vi "Read Spectrum Continuously.vi"() -> ()   [LabVIEW 2021]
uses:
  <vilib>/Utility/error.llb/DialogType.ctl
panel:
  out "Spectrum number":i32
  out "Read time (ms)":u32
  in  "Ref Level Auto":bool
  out "Min":dbl
  out "Sec":dbl
  out "H":dbl
  in  "Stop Button":bool
  out "P x Lambda Graph":cluster{dbl[], dbl[]}(graph)
  out "Corrente Atual (mA)":dbl
  out "P x I Graph":cluster{dbl[], dbl[]}(graph)
  in  "Start Button":bool
  in  "Cluster de Dados de Entrada":T1={"Corrente Inicial (mA)"=150.0, "Limite de Temperatura"=27.0, "Temperatura"=25.0, "Corrente Limite (mA)"=300, "Centralizar pico (nm)"=1550.0, "Valor de Span (nm)"=200.0, "Passo (mA)"=0.0, "Corrente Final (mA)"=150.0, "Resolucao"=enum."High", "Modo"=enum."Laser"} {"Corrente Final (mA)" min=0.0 step=1.0; "Passo (mA)" min=1.0 step=1.0; "Valor de Span (nm)" min=0.1 max=1400.0 format="%.2f"; "Centralizar pico (nm)" format="%.2f"; "Temperatura" min=-100.0 max=199.9 step=0.1; "Limite de Temperatura" min=-100.0 max=199.9 step=0.1; "Corrente Inicial (mA)" min=0.0 step=1.0}
  out "XY Graph":T2(graph)
  in  "Pasta Destino":path=path "d:/Users/acquisition"
  in  "GPIB Analisador de Espectros":refnum<visa-resource-name>="GPIB0::8::INSTR"
  in  "error in (no error)":errorcluster
  out "error out":errorcluster
  # "Tempo Gasto"
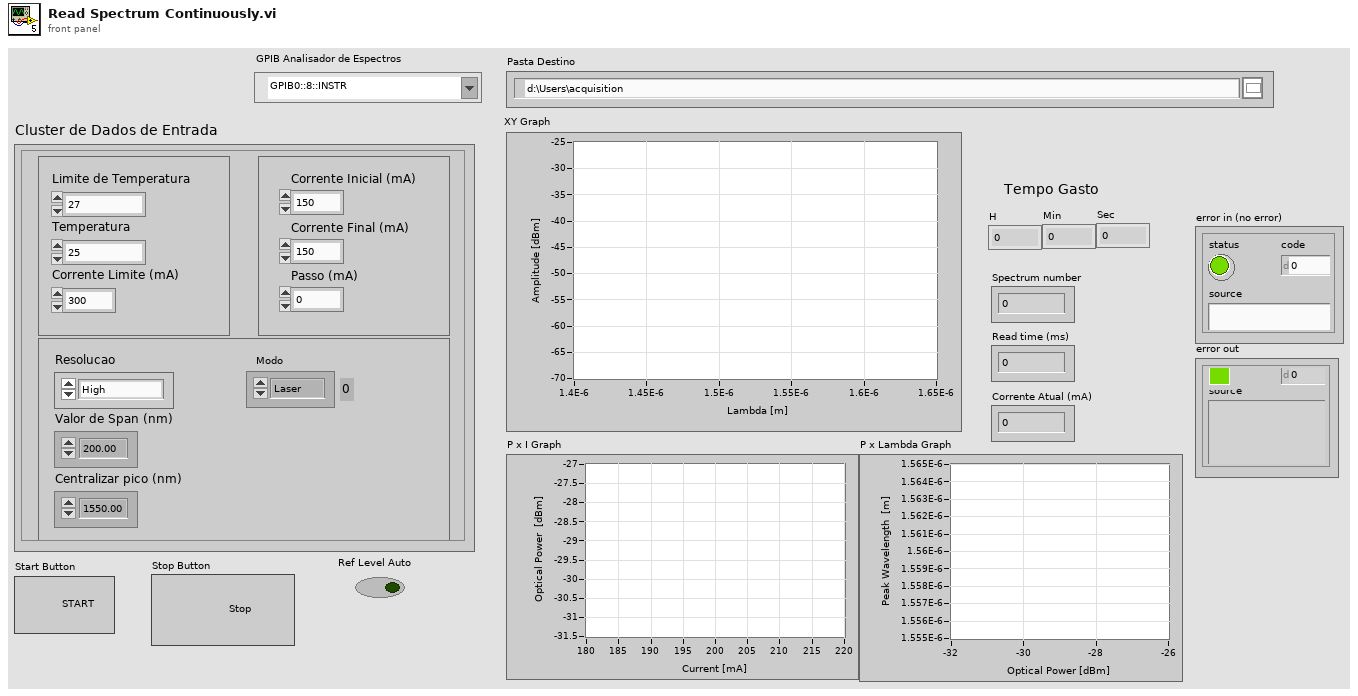
[diagram p1: front panel]
types:
  T1 = cluster{"Corrente Inicial (mA)":dbl, "Limite de Temperatura":dbl, "Temperatura":dbl, "Corrente Limite (mA)":i32, "Centralizar pico (nm)":dbl, "Valor de Span (nm)":dbl, "Passo (mA)":dbl, "Corrente Final (mA)":dbl, "Resolucao":enum16{"Normal", "High"}, "Modo":enum16{"Laser", "Led"}}
  T2 = cluster{"Wavelike Data":dbl[], "Wavelike Data":dbl[]}
  T3 = typedef "DialogType.ctl" = u16
  T4 = cluster{"Limite de Temperatura":dbl, "Temperatura":dbl, "Corrente Inicial (mA)":dbl, "Corrente Limite (mA)":i32, "Resolucao":enum16{"Normal", "High"}, "Centralizar pico (nm)":dbl, "Valor de Span (nm)":dbl, "Modo":enum16{"Laser", "Led"}}
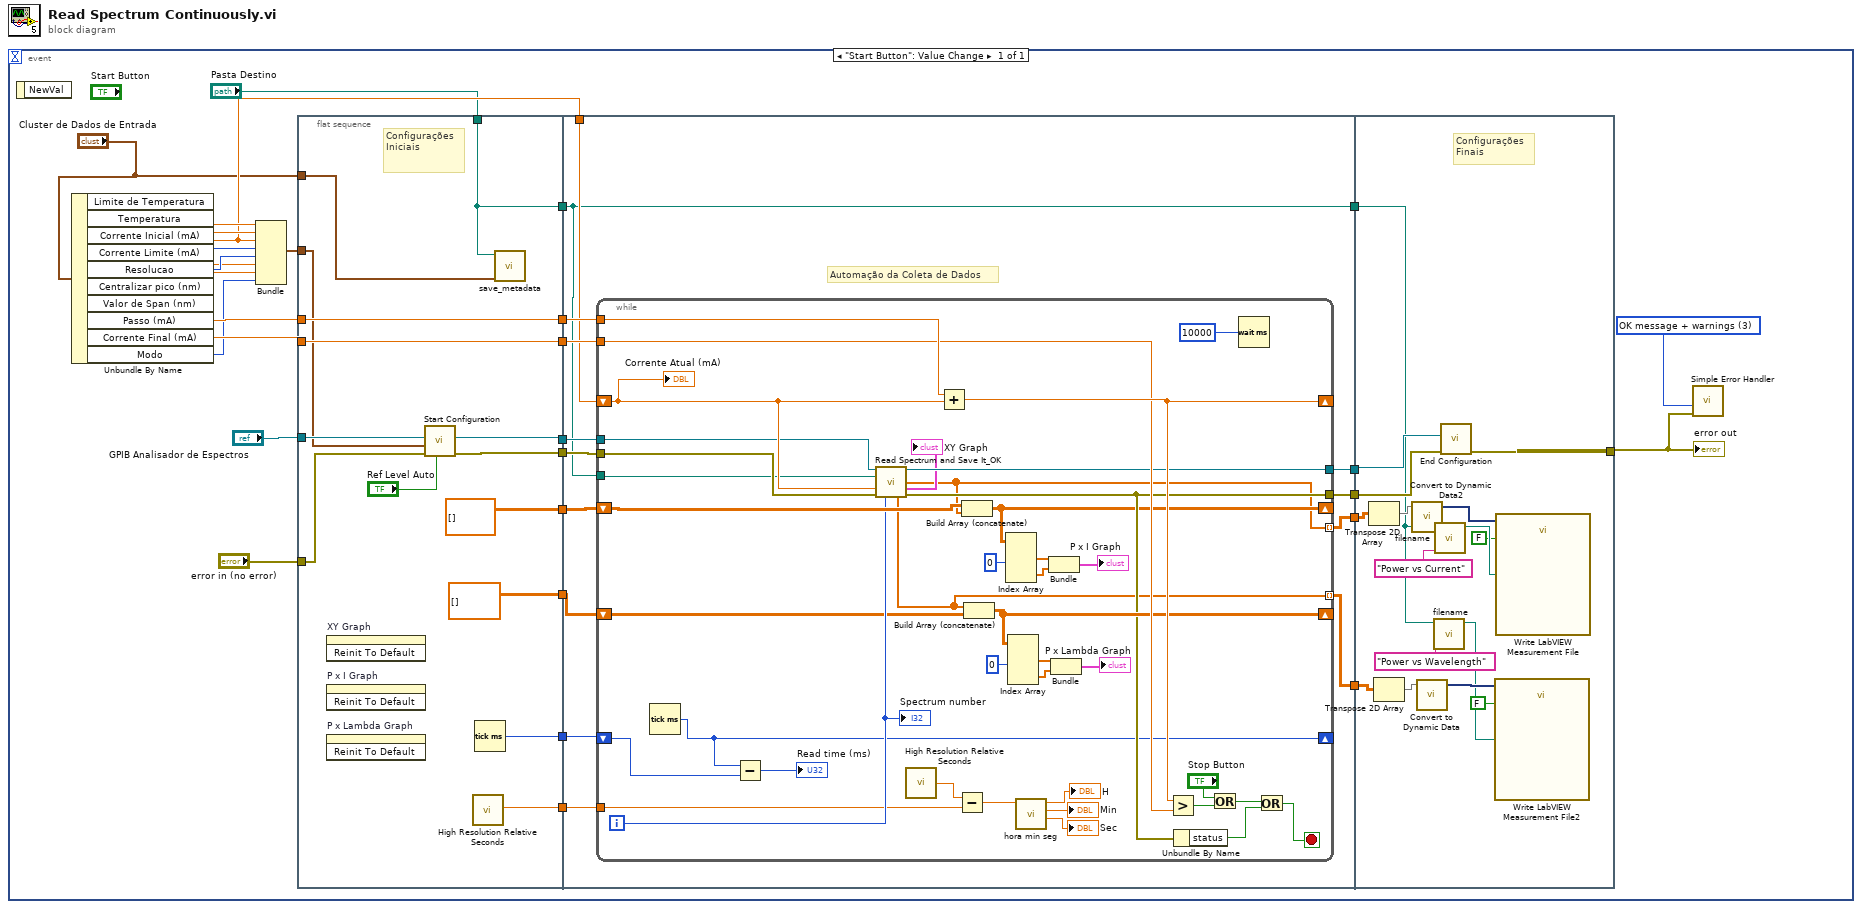
[diagram p0: block diagram]
diagram:
  n1 = event shown="[0] \"Start Button\": Value Change" {
    selector: _ -> [_]
    dyn-events: _ -> [_]
    timeout: _ -> [_]
    event "Start Button": Value Change {
      w11 = T3 3 items=["no dialog", "OK message", "continue or stop message", "OK message + warnings", "continue/stop + warnings"] ("type of dialog (OK msg:1)")
      n2 = event-data() -> ()  [unwired: 1 in, 1 out]
      n3 = Unbundle By Name("Cluster de Dados de Entrada") -> ("Limite de Temperatura"=w25:dbl, "Temperatura"=w24:dbl, "Corrente Inicial (mA)"=w16:dbl, "Corrente Limite (mA)"=w23:i32, "Resolucao"=w22:enum16{"Normal", "High"}, "Centralizar pico (nm)"=w21:dbl, "Valor de Span (nm)"=w19:dbl, "Passo (mA)"=w18:dbl, "Corrente Final (mA)"=w17:dbl, "Modo"=w5:enum16{"Laser", "Led"})
      n4 = Bundle("Limite de Temperatura"=w25, "Temperatura"=w24, "Corrente Inicial (mA)"=w16, "Corrente Limite (mA)"=w23, "Resolucao"=w22, "Centralizar pico (nm)"=w21, "Valor de Span (nm)"=w19, "Modo"=w5) -> (w20:T4)  [unwired: 1 in]
      n5 = flat-sequence {
        tunnel: "error in (no error)" -> [w39]
        tunnel: [w45] -> w31
        tunnel: "GPIB Analisador de Espectros" -> [w44]
        tunnel: [w43] -> w30
        tunnel: [w42] -> w29
        tunnel: w18 -> [w42]
        tunnel: w17 -> [w41]
        tunnel: [w41] -> w28
        tunnel: w20 -> [w36]
        tunnel: [dbl[][] []] -> w15
        tunnel: [dbl[][] []] -> w10
        tunnel: "Cluster de Dados de Entrada" -> [w33]
        tunnel: [w35] -> w4
        tunnel: [w34] -> w3
        tunnel: [w32] -> w2
        tunnel: "Pasta Destino" -> [w32]
        tunnel: w31 -> [w59]
        tunnel: w30 -> [w58]
        tunnel: w29 -> [w57]
        tunnel: w28 -> [w56]
        tunnel: w16 -> [w55]
        tunnel: w15 -> [w54]
        tunnel: [w53] -> w14
        tunnel: [w52] -> w13
        tunnel: w10 -> [w51]
        tunnel: [w46] -> w9
        tunnel: [w50] -> w8
        tunnel: [w49] -> w7
        tunnel: w4 -> [w48]
        tunnel: w3 -> [w47]
        tunnel: w2 -> [w46]
        tunnel: [w115] -> w12
        tunnel: w14 -> [w114]
        tunnel: w13 -> [w113]
        tunnel: w9 -> [w102]
        tunnel: w8 -> [w104]
        tunnel: w7 -> [w106]
        frame #0 {
          # "Configurações\nIniciais"
          n6 = invoke on="XY Graph" class="XYGraph (strict)" method="Reinit To Default"() -> ()  [unwired: 3 in, 3 out]
          n7 = invoke on="P x I Graph" class="XYGraph (strict)" method="Reinit To Default"() -> ()  [unwired: 3 in, 3 out]
          n8 = invoke on="P x Lambda Graph" class="XYGraph (strict)" method="Reinit To Default"() -> ()  [unwired: 3 in, 3 out]
          n9 = call "Start Configuration.vi"("Ref Lvl Auto"="Ref Level Auto", "error in (no error)"=w39, "Cluster de Dados"=w36, "GPIB Espectrometro"=w44) -> ("error out"=w45:errorcluster, "Spectrometer out"=w43:refnum<visa-resource-name>)  [unwired: 6 in]
          n10 = call <vilib>:"High Resolution Relative Seconds.vi"() -> ("relative seconds"=w34:dbl)
          n11 = Tick Count (ms)() -> (millisecond timer value=w35:u32)
          n12 = call "save_metadata.vi"("Cluster de Dados de Entrada"=w33, "Pasta Destino"=w32) -> ()  [unwired: 10 in]
        }
        frame #1 {
          # "Automação da Coleta de Dados"
          n13 = while {
            shift-right: [w97] -> _
            shift-left: w55 -> [w98]
            tunnel: w59 -> [w91]
            tunnel: w58 -> [w96]
            tunnel: w57 -> [w95]
            tunnel: w56 -> [w94]
            shift-right: [w69] -> _
            shift-left: w54 -> [w90]
            tunnel: [w79] -> w53
            tunnel: [w85] -> w52
            shift-right: [w80] -> _
            shift-left: w51 -> [w81]
            tunnel: w46 -> [w70]
            tunnel: [w68] -> w50 mode=indexing
            tunnel: [w67] -> w49 mode=indexing
            shift-right: [w64] -> _
            shift-left: w48 -> [w66]
            tunnel: w47 -> [w62]
            i -> [w86]
            stop <- w77 stop-if-true
            n14 = Tick Count (ms)() -> (millisecond timer value=w64:u32)
            n15 = Subtract(x=w64, y=w66) -> (x-y=→"Read time (ms)":u32)
            n16 = call "Read Spectrum and Save It_OK.vi"("VISA Session"=w96, "Pasta Destino DESTA aquisicao"=w70, "Corrente Atual (mA)"=w98, "Error In"=w91, "Iteracao"=w86) -> ("Copy VISA Session"=w85:refnum<visa-resource-name>, "PxI"=w67:dbl[], "XY Graph"=→"XY Graph":T2, "PxLambda"=w68:dbl[], "Error Out"=w79:errorcluster)  [unwired: 4 in, 2 out]
            n17 = call <vilib>:"High Resolution Relative Seconds.vi"() -> ("relative seconds"=w63:dbl)
            n18 = Add(x=w95, y=w98) -> (x+y=w97:dbl)
            n19 = Subtract(x=w63, y=w62) -> (x-y=w61:dbl)
            n20 = Build Array (concatenate)(w90, w67) -> (w69:dbl[][])
            n21 = Build Array (concatenate)(w68, w81) -> (w80:dbl[][])
            n22 = Index Array(array=w69, index (col) #1=0 ("disabled index (col)")) -> (element #1=w88:dbl[], element #2=w87:dbl[])  [unwired: 3 in]
            n23 = Index Array(array=w80, index (col) #1=0 ("disabled index (col)")) -> (element #1=w83:dbl[], element #2=w82:dbl[])  [unwired: 3 in]
            n24 = call "hora min seg.vi"("Total time in seconds"=w61) -> ("Sec"=→"Sec":dbl, "Min"=→"Min":dbl, "H"=→"H":dbl)  [unwired: 8 in]
            n25 = Bundle(w88, w87) -> (→"P x I Graph":cluster{dbl[], dbl[]})  [unwired: 1 in]
            n26 = Bundle(w83, w82) -> (→"P x Lambda Graph":cluster{dbl[], dbl[]})  [unwired: 1 in]
            n27 = Greater?(x=w97, y=w94) -> (0:w99:bool)
            n28 = Unbundle By Name(w79) -> ("status"=w92:bool)
            n29 = Or(x="Stop Button", y=w99) -> (x .or. y?=w93:bool)
            n30 = Wait (ms)(milliseconds to wait=u32 10000 ("millisecond multiple")) -> ()  [unwired: 1 out]
            n31 = Or(x=w93, y=w92) -> (x .or. y?=w77:bool)
            "Corrente Atual (mA)" <- w98
            "Spectrum number" <- w86
          }
        }
        frame #2 {
          # "Configurações\nFinais"
          n32 = Transpose 2D Array(2D array=w106) -> (transposed array=w105:dbl[][])
          n33 = Transpose 2D Array(2D array=w104) -> (transposed array=w103:dbl[][])
          n34 = call "Convert to Dynamic Data2"("2D Array"=w105) -> ("Dynamic Data Type"=w109:dynamicdata)  [unwired: 3 in]
          n35 = call "Convert to Dynamic Data"("2D Array"=w103) -> ("Dynamic Data Type"=w110:dynamicdata)  [unwired: 3 in]
          n36 = call "filename.vi"("Filename"="Power vs Wavelength", "Pasta Destino"=w102) -> ("filename output"=w107:path)  [unwired: 9 in]
          n37 = call "filename.vi"("Filename"="Power vs Current", "Pasta Destino"=w102) -> ("filename output"=w108:path)  [unwired: 9 in]
          n38 = call "End Configuration.vi"("error in (no error)"=w114, "GPIB Espectrometro"=w113) -> ("error out"=w115:errorcluster)  [unwired: 9 in]
          n39 = call "Write LabVIEW Measurement File2"("Signals"=w110, "Enable"=FALSE, "Filename"=w107) -> ()  [unwired: 14 in, 3 out]
          n40 = call "Write LabVIEW Measurement File"("Signals"=w109, "Enable"=FALSE, "Filename"=w108) -> ()  [unwired: 14 in, 3 out]
        }
      }
      n41 = call <vilib>:"Simple Error Handler.vi"("type of dialog (OK msg:1)"=w11, "error in (no error)"=w12) -> ()  [unwired: 3 in, 5 out]
      "error out" <- w12
    }
  }
